vi "往复运动.vi"(6 "停止模式":enum32{"Dec", "Emg"}(ring), 9 "AxisHandle":u32, 10 "设置速度":dbl, 11 "设定距离":dbl) -> ()   [LabVIEW 2016]
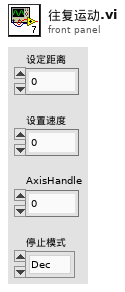
[diagram p1: front panel]
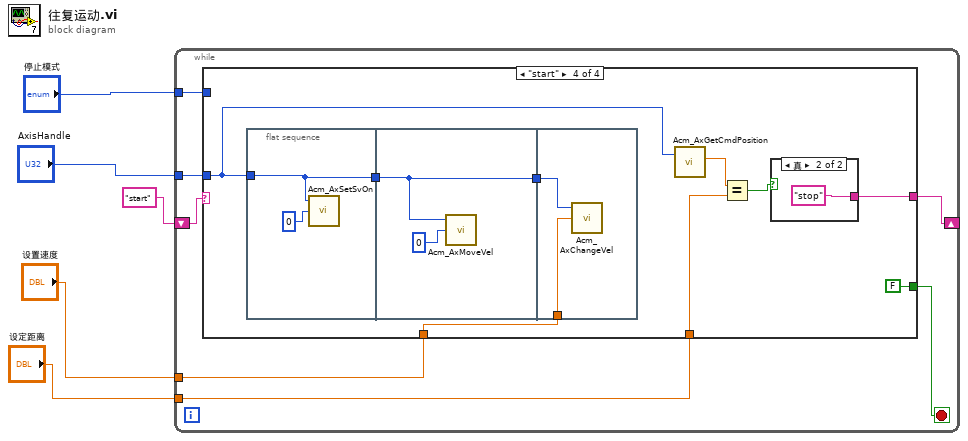
[diagram p0: block diagram]
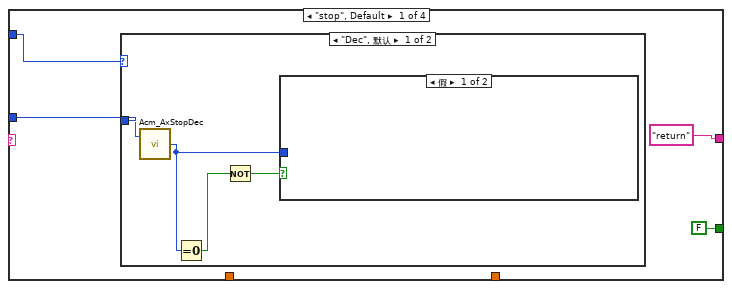
[diagram p2: hidden frame]
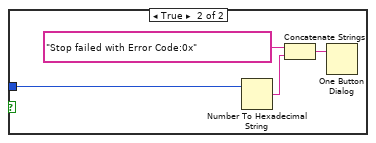
[diagram p3: hidden frame]
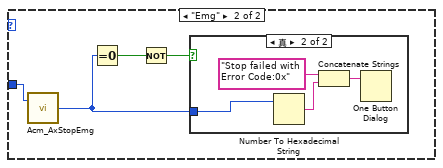
[diagram p4: hidden frame]
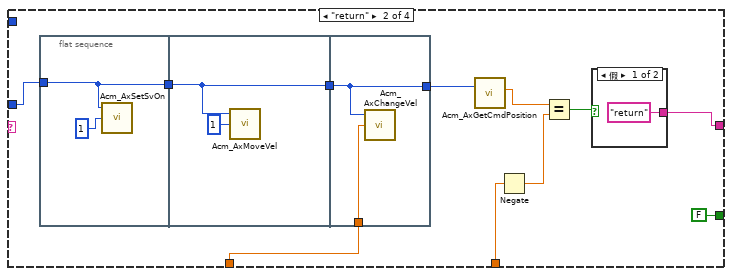
[diagram p6: hidden frame]
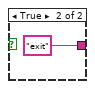
[diagram p7: hidden frame]
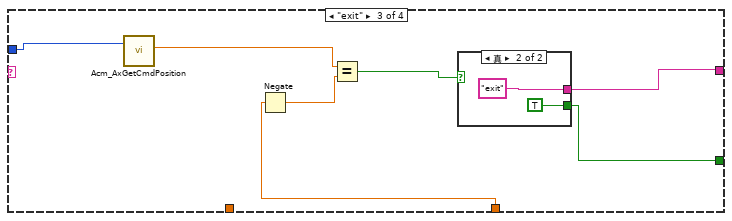
[diagram p8: hidden frame]
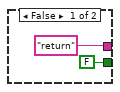
[diagram p9: hidden frame]
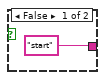
[diagram p10: hidden frame]
diagram:
  n1 = while {
    tunnel: "AxisHandle" -> [w12]
    shift-right: [w10] -> _
    shift-left: "start" -> [w11]
    tunnel: "设置速度" -> [w8]
    tunnel: "设定距离" -> [w7]
    tunnel: "停止模式" -> [w6]
    stop <- w9 stop-if-true
    n2 = case shown="\"start\"" w11 {
      tunnel: w12 -> [w16 w41 w57 w66]
      tunnel: w8 -> [_ w40 _ w69]
      tunnel: w7 -> [_ w33 w54 w68]
      tunnel: ["return" w39 w55 w64] -> w10
      tunnel: [FALSE FALSE w52 FALSE] -> w9
      tunnel: w6 -> [w13 _ _ _]
      frame "stop", Default {
        n3 = case shown="\"Dec\", 默认" w13 {
          tunnel: w16 -> [w20 w28]
          frame "Dec", Default {
            n4 = call <userlib>:"Acm_AxStopDec.vi"("AxisHandle"=w20) -> ("ReturnValue"=w19:u32)  [unwired: 1 in, 2 out]
            n5 = Equal To 0?(x=w19) -> (x = 0?=w18:bool)
            n6 = Not(x=w18) -> (.not. x?=w17:bool)
            n7 = case shown="假" w17 {
              tunnel: w19 -> [_ w24]
              frame False {
              }
              frame True {
                n8 = Number To Hexadecimal String(2:w24) -> (0:w22:string)  [unwired: 1 out]
                n9 = Concatenate Strings("Stop failed with Error Code:0x", w22) -> (w21:string)
                n10 = One Button Dialog(message=w21) -> ()  [unwired: 2 out]
              }
            }
          }
          frame "Emg" {
            n11 = call <userlib>:"Acm_AxStopEmg.vi"("AxisHandle"=w28) -> ("ReturnValue"=w27:u32)  [unwired: 1 in, 2 out]
            n12 = Equal To 0?(x=w27) -> (x = 0?=w26:bool)
            n13 = Not(x=w26) -> (.not. x?=w25:bool)
            n14 = case shown="真" w25 {
              tunnel: w27 -> [_ w32]
              frame False {
              }
              frame True {
                n15 = Number To Hexadecimal String(2:w32) -> (0:w30:string)  [unwired: 1 out]
                n16 = Concatenate Strings("Stop failed with Error Code:0x", w30) -> (w29:string)
                n17 = One Button Dialog(message=w29) -> ()  [unwired: 2 out]
              }
            }
          }
        }
      }
      frame "return" {
        n18 = flat-sequence {
          tunnel: w41 -> [w46]
          tunnel: [w46] -> w43
          tunnel: w43 -> [w48]
          tunnel: [w48] -> w42
          tunnel: w42 -> [w50]
          tunnel: w40 -> [w51]
          tunnel: [w50] -> w36
          frame #0 {
            n19 = call <userlib>:"Acm_AxSetSvOn.vi"("OnOff"=u32 1, "AxisHandle"=w46) -> ()  [unwired: 1 in, 3 out]
          }
          frame #1 {
            n20 = call <userlib>:"Acm_AxMoveVel.vi"("Direction"=u16 1, "AxisHandle"=w48) -> ()  [unwired: 1 in, 3 out]
          }
          frame #2 {
            n21 = call <userlib>:"Acm_AxChangeVel.vi"("NewVelocity"=w51, "AxisHandle"=w50) -> ()  [unwired: 1 in, 3 out]
          }
        }
        n22 = call <userlib>:"Acm_AxGetCmdPosition.vi"("AxisHandle"=w36) -> ("Position"=w37:dbl)  [unwired: 1 in, 3 out]
        n23 = Negate(x=w33) -> (-x=w34:dbl)
        n24 = Equal?(x=w37, y=w34) -> (x = y?=w35:bool)
        n25 = case shown="假" w35 {
          tunnel: ["return" "exit"] -> w39
          frame False {
          }
          frame True {
          }
        }
      }
      frame "exit" {
        n26 = call <userlib>:"Acm_AxGetCmdPosition.vi"("AxisHandle"=w57) -> ("Position"=w58:dbl)  [unwired: 1 in, 3 out]
        n27 = Negate(x=w54) -> (-x=w53:dbl)
        n28 = Equal?(x=w58, y=w53) -> (x = y?=w56:bool)
        n29 = case shown="真" w56 {
          tunnel: ["return" "exit"] -> w55
          tunnel: [FALSE TRUE] -> w52
          frame False {
          }
          frame True {
          }
        }
      }
      frame "start" {
        n30 = flat-sequence {
          tunnel: w66 -> [w74]
          tunnel: [w74] -> w71
          tunnel: w71 -> [w76]
          tunnel: [w76] -> w70
          tunnel: w70 -> [w79]
          tunnel: w69 -> [w78]
          frame #0 {
            n31 = call <userlib>:"Acm_AxSetSvOn.vi"("OnOff"=u32 0, "AxisHandle"=w74) -> ()  [unwired: 1 in, 3 out]
          }
          frame #1 {
            n32 = call <userlib>:"Acm_AxMoveVel.vi"("Direction"=u16 0, "AxisHandle"=w76) -> ()  [unwired: 1 in, 3 out]
          }
          frame #2 {
            n33 = call <userlib>:"Acm_AxChangeVel.vi"("NewVelocity"=w78, "AxisHandle"=w79) -> ()  [unwired: 1 in, 3 out]
          }
        }
        n34 = call <userlib>:"Acm_AxGetCmdPosition.vi"("AxisHandle"=w66) -> ("Position"=w67:dbl)  [unwired: 1 in, 3 out]
        n35 = Equal?(x=w67, y=w68) -> (x = y?=w65:bool)
        n36 = case shown="真" w65 {
          tunnel: ["start" "stop"] -> w64
          frame False {
          }
          frame True {
          }
        }
      }
    }
  }
